vi "Close.vi"(8 "error in":errorcluster, 11 "UserEventHandler in":refnum<class "UserEventHandler.lvclass">) -> (0 "error out":errorcluster, 3 "UserEventHandler out":refnum<class "UserEventHandler.lvclass">)   [LabVIEW 2024, in "hse-logger.lvlib" / "UserEventHandler.lvclass"]
doc: "Destroys the user event. This method should be called when the ``Logger`` gets closed or the handler is removed from the ``Logger``.\n\n____\nHAMPEL SOFTWARE ENGINEERING v2.2.2 (2025-01-16 15:41)"
uses:
  <vilib>/Hampel Software Engineering/HSE Logger/Handler/UserEventHandler/UserEventHandler.lvclass
  <vilib>/Hampel Software Engineering/HSE Logger/Handler/UserEventHandler/UserEventHandler.lvclass/UserEventHandler.ctl
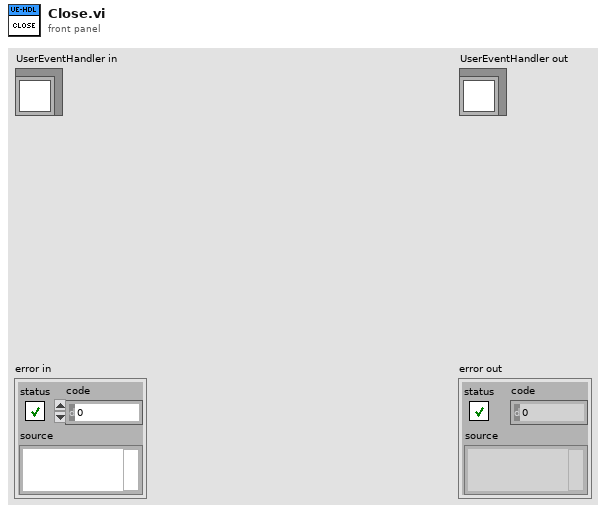
[diagram p1: front panel]
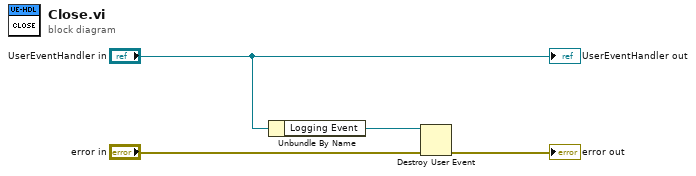
[diagram p0: block diagram]
diagram:
  n1 = Unbundle By Name("UserEventHandler in") -> ("Logging Event"=w1:refnum<user-event>)
  n2 = Destroy User Event(user event=w1, error in="error in") -> (error out=→"error out":errorcluster)
  "UserEventHandler out" <- "UserEventHandler in"
